vi "RMS (1 Channel).vi"(8 "error in (no error)":errorcluster, 11 "waveform":waveform(dbl)) -> (0 "error out":errorcluster, 3 "RMS value":dbl)   [LabVIEW 2013, in "NI_EP_Basic.lvlib"]
doc: "Calculates the RMS level of a voltage or current signal. Wire data to the <B>waveform</B> input to determine the polymorphic instance to use or manually select the instance."
uses:
  <vilib>/addons/Electrical Power/Basic/NI_EP_Basic.lvlib
  <vilib>/Analysis/5stat.llb/RMS (DBL).vi
  <vilib>/Analysis/NI_AALPro.lvlib
  <vilib>/measure/NI_MABase.lvlib
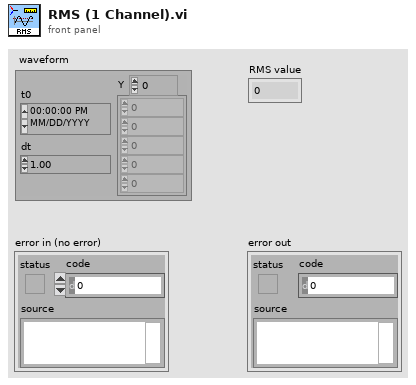
[diagram p1: front panel]
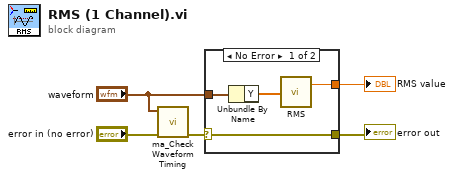
[diagram p0: block diagram]
diagram:
  n1 = call <vilib>:"ma_Check Waveform Timing.vi"("error in (no error)"="error in (no error)", "signal in"="waveform") -> ("error out"=w2:errorcluster)  [unwired: 1 in, 8 out]
  n2 = case shown="No Error" w2 {
    selector: w2 -> [w6 w10]
    tunnel: [w9 _] -> w5
    tunnel: [w6 w10] -> w4
    tunnel: "waveform" -> [w8 _]
    frame No Error {
      n3 = Unbundle By Name(w8) -> ("Y"=w7:dbl[])
      n4 = call-poly <vilib>:"RMS.vi"("X"=w7) -> ("rms value"=w9:dbl)  [unwired: 1 out]
    }
    frame Error {
    }
  }
  "RMS value" <- w5
  "error out" <- w4
